vi "Pack Mission Upload Message.vi"(11 "Test Mission":T1[](array[typedef]) {"GPS Longitude" format="%.6g"; "GPS Latitude" format="%.6g"}) -> (3 "Mission Upload Message out":refnum<class "Mission Upload Message.lvclass">)   [LabVIEW 2015, in "RDS Mission Controller Actor.lvlib"]
uses:
  RDS Mission Controller Actor.lvlib
  Libraries/RDS Child Messages/Mission Messages/Mission Upload Message.lvclass
  MissionOp.ctl
  Libraries/RDS Framework/RDS Message ID.ctl
  Libraries/RDS Framework/RDS Message Class/RDS Message.lvclass/RDS Message.ctl
  Libraries/RDS Child Messages/Mission Messages/Mission Upload Message.lvclass/Mission Upload Message.ctl
  Libraries/RDS Framework/RDS Message Class/RDS Message.lvclass
  Libraries/RDS Child Messages/RDS Child Messages.lvlib
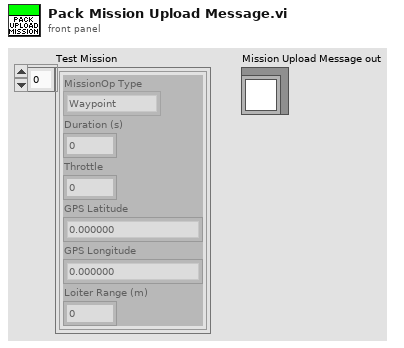
[diagram p1: front panel]
types:
  T1 = typedef "RDS Mission Controller Actor.lvlib/MissionOp.ctl" = cluster{"MissionOp Type":enum16{"Waypoint", "Loiter", "Wait", "Deploy AIP", "Stow AIP"}, "Duration (s)":u16, "Throttle":i16, "GPS Latitude":dbl, "GPS Longitude":dbl, "Loiter Range (m)":u16}
  T2 = typedef "RDS Child Messages.lvlib/RDS Message ID.ctl" = enum16{"RDS Hello World", "String Message", "AIP_Status", "AIP_Command", "GPS_Data", "MCB_Command", "MCB_Status", "Compass_Data", "Depth_Data", "Battery_Data", "Contoller_State", "Set_Mag_Dev", "BTB_Shutdown", "State_Sample_Request", "State_Sample", "PID_Gains_Set", "Helm_Limiter_Set", "Helm_Heading_Command", "Helm_Steering_Command", "Helm_Status", "Controller_Message", "AIP_Set_Min_Depth", "Mission_Controller_State", "Mission_Upload", "Mission_Set_Op_and_Run", "Mission_Settings_Set"}
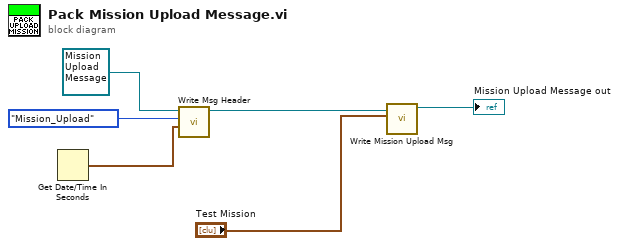
[diagram p0: block diagram]
diagram:
  n1 = Get Date/Time In Seconds() -> (seconds since 1Jan1904=w3:timestamp)
  n2 = call "Write Msg Header.vi"("Time Stamp"=w3, "Msg ID"=RDS_Message_ID."Mission_Upload", "RDS Message in"=refnum<class "Mission Upload Message.lvclass"> refnum ("RDS Child Messages.lvlib:Mission Upload Message.lvclass")) -> ("RDS Message out"=w4:refnum<class "Mission Upload Message.lvclass">)  [unwired: 7 in, 1 out]
  n3 = call "Write Mission Upload Msg.vi"("Mission"="Test Mission", "Load Mission Message in"=w4) -> ("Load Mission Message out"=→"Mission Upload Message out":refnum<class "Mission Upload Message.lvclass">)  [unwired: 8 in, 1 out]
